vi "Configure Frequency Sweep.vi"(0 "VISA resource name":refnum<visa-resource-name>, 1 "Sweep Direction (0: Up)":u16(ring) items=["Up", "Down", "Up/Down", "Down/Up"], 2 "Sweep Marker (100 Hz)":dbl=100.0, 5 "Sweep Type (0: Continuous)":u16(ring) items=["Continuous", "Triggered", "Triggered, Hold/Reset"], 7 "Sweep Spacing (0: Linear)":u16(ring) items=["Linear", "Log"], 9 "Sweep Time (1.00 s)":dbl=1.0 format="%#.6g", 11 "error in (no error)":errorcluster, 12 "Start Frequency (100.0 Hz)":dbl=100.0 format="%#.6g", 13 "Stop  Frequency  (1000.0 Hz)":dbl=1000.0 format="%#.6f") -> (4 "VISA resource name out":refnum<visa-resource-name>, 15 "error out":errorcluster)   [LabVIEW 2015, in "Fluke 28x Series.lvlib"]
doc: "Configures and enables a frequency sweep. In the frequency sweep mode, the function generator steps from the start frequency to the stop frequency at a sweep rate."
uses:
  <instrlib>/Fluke 28x Series/Fluke 28x Series.lvlib
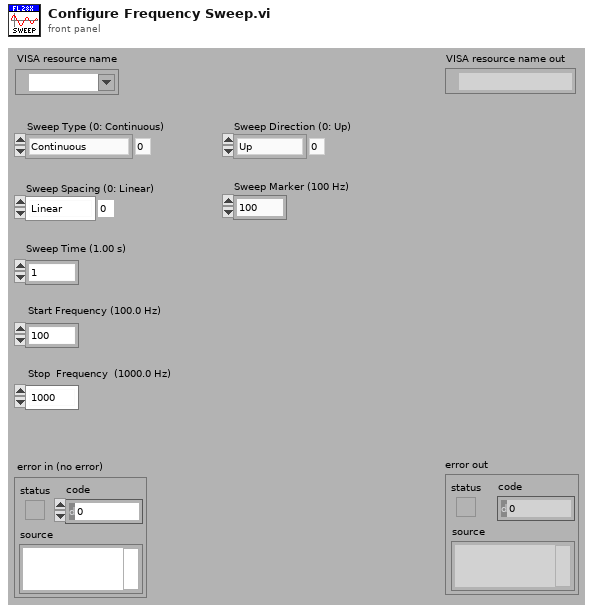
[diagram p1: front panel]
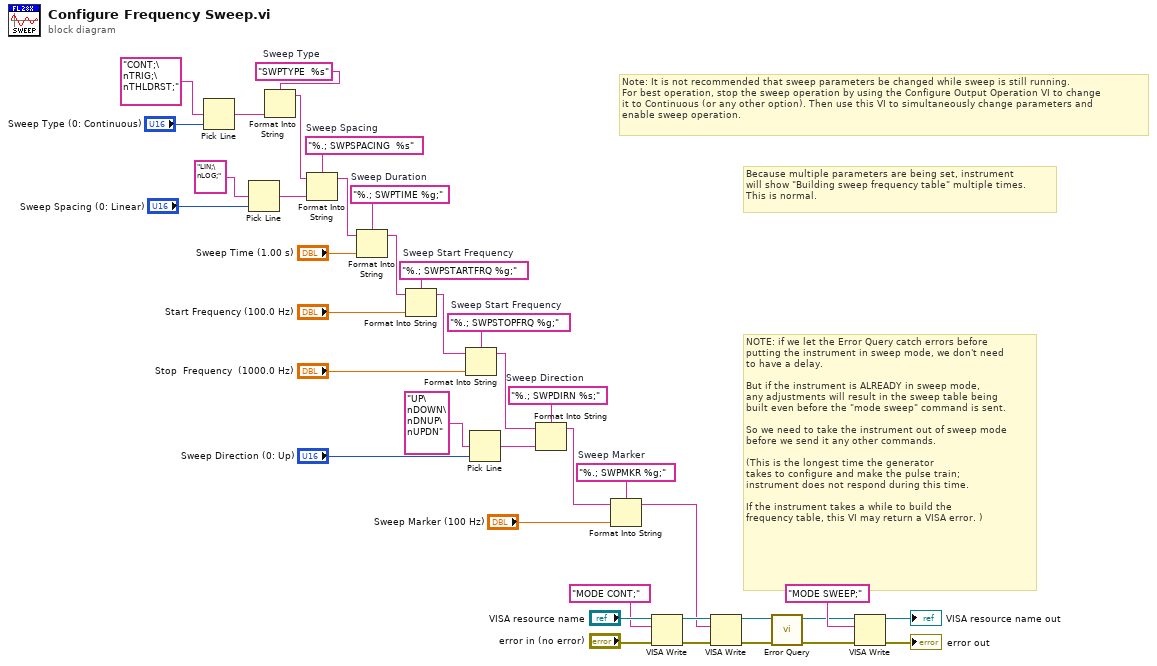
[diagram p0: block diagram]
diagram:
  w16 = "%.; SWPMKR %g;"  # Sweep Marker
  w19 = "%.; SWPDIRN %s;"  # Sweep Direction
  w24 = "SWPTYPE  %s"  # Sweep Type
  w32 = "%.; SWPSTOPFRQ %g;"  # Sweep Start Frequency
  w34 = "%.; SWPSTARTFRQ %g;"  # Sweep Start Frequency
  w37 = "%.; SWPTIME %g;"  # Sweep Duration
  w31 = "%.; SWPSPACING  %s"  # Sweep Spacing
  # "Note: It is not recommended that sweep parameters be changed while sweep is still running.\nFor best operation, stop the sweep operation by using the Configure Output Operation VI to change\nit to Continuous (or any other option). Then use this VI to simultaneously change parameters and \nenable sweep operation."
  # "Because multiple parameters are being set, instrument\nwill show \"Building sweep frequency table\" multiple times.\nThis is normal."
  # "NOTE: if we let the Error Query catch errors before \nputting the instrument in sweep mode, we don't need \nto have a delay.\n\nBut if the instrument is ALREADY in sweep mode,\nany adjustments will result in the sweep table being\nbuilt even before the \"mode sweep\" command is sent. \n\nSo we need to take the instrument out of sweep mode\nbefore we send it any other commands. \n\n(This is the longest time the generator\ntakes to configure and make the pulse train;\ninstrument does not respond during this time.\n\nIf the instrument takes a while to build the \nfrequency table, this VI may return a VISA error. )"
  n1 = Pick Line(multi-line string="CONT;\nTRIG;\nTHLDRST;", line index="Sweep Type (0: Continuous)") -> (output string=w17:string)  [unwired: 1 in]
  n2 = Pick Line(multi-line string="LIN;\nLOG;", line index="Sweep Spacing (0: Linear)") -> (output string=w30:string)  [unwired: 1 in]
  n3 = Format Into String(format string=w24, w17) -> (resulting string=w23:string)  [unwired: 2 in, 1 out]
  n4 = Format Into String(format string=w31, initial string=w23, w30) -> (resulting string=w29:string)  [unwired: 1 in, 1 out]
  n5 = Format Into String(format string=w37, initial string=w29, "Sweep Time (1.00 s)") -> (resulting string=w36:string)  [unwired: 1 in, 1 out]
  n6 = Format Into String(format string=w34, initial string=w36, "Start Frequency (100.0 Hz)") -> (resulting string=w33:string)  [unwired: 1 in, 1 out]
  n7 = Format Into String(format string=w32, initial string=w33, "Stop  Frequency  (1000.0 Hz)") -> (resulting string=w18:string)  [unwired: 1 in, 1 out]
  n8 = Pick Line(multi-line string="UP\nDOWN\nDNUP\nUPDN", line index="Sweep Direction (0: Up)") -> (output string=w20:string)  [unwired: 1 in]
  n9 = Format Into String(format string=w19, initial string=w18, w20) -> (resulting string=w14:string)  [unwired: 1 in, 1 out]
  n10 = Format Into String(format string=w16, initial string=w14, "Sweep Marker (100 Hz)") -> (resulting string=w1:string)  [unwired: 1 in, 1 out]
  n11 = VISA Write(VISA resource name="VISA resource name", write buffer="MODE CONT;", error in (no error)="error in (no error)") -> (VISA resource name out=w5:refnum<visa-resource-name>, error out=w6:errorcluster)  [unwired: 1 out]
  n12 = VISA Write(VISA resource name=w5, write buffer=w1, error in (no error)=w6) -> (VISA resource name out=w13:refnum<visa-resource-name>, error out=w12:errorcluster)  [unwired: 1 out]
  n13 = call <instrlib>:"Error Query.vi"("error in (no error)"=w12, "VISA resource name"=w13) -> ("error out"=w9:errorcluster, "VISA resource name out"=w10:refnum<visa-resource-name>)  [unwired: 6 in, 2 out]
  n14 = VISA Write(VISA resource name=w10, write buffer="MODE SWEEP;" ("string"), error in (no error)=w9) -> (VISA resource name out=→"VISA resource name out":refnum<visa-resource-name>, error out=→"error out":errorcluster)  [unwired: 1 out]
